vi "0805_Visão_de_máquina.vi"() -> ()   [LabVIEW 2017]
uses:
  <vilib>/userdefined/High Color/IMAQdx.ctl
  <vilib>/vision/driver/IMAQdx.llb/IMAQdx Acquisition Mode.ctl
  <vilib>/vision/driver/IMAQdx.llb/IMAQdx Buffer Number Mode.ctl
  <vilib>/vision/Classification.llb/IMAQ Classifier Read Options.ctl
  <vilib>/vision/driver/NI_Vision_Acquisition_Software.lvlib
  <vilib>/vision/NI_Vision_Development_Module.lvlib
panel:
  out "Array de classes":string[](array[string])
  out "Array de pos":string[](array[string])
  out "Array (0)":string[](array[string])
  out "Peça a ser manufatruada(0)":string[](array[string])
  out "Peça a ser manufatruada":string[](array[string])
  in  "Peça a ser manufaturada":T1
  out "x .and. y? 2":bool
  out "x = y? 2":bool
  out "x = y?":bool
  out "Boolean 2":bool
  out "concatenated string 3":string
  out "seletou_detectou":bool
  in  "Comunicação de dados":bool
  out "concatenated string 2":string
  out "concatenated string":string
  out "Boolean":bool
  out "Parar_esteira":bool
  out "aux":bool
  out "normal":u32
  out "parou":u32
  out "detectou":u32
  out "Detectou":bool
  out "reconheceu":bool
  out "bool_parou":bool
  out "bool_normal":bool
  out "bool_detectou":bool
  out "reconhecendo":bool
  out "Stop 3":bool
  out "seletor":enum16{"normal", "detectou", "parou"}(ring)=enum."detectou"
  in  "enum":enum16{"normal", "detectou", "parou"}(ring)=enum."detectou"
  out "x .and. y?":bool
  in  "dimensão_x_ROI_esteira":sgl=30.0
  in  "dimensão_y_ROI_esteira":sgl=30.0
  in  "posicao_y_ROI_esteira":sgl
  in  "posicao_x_ROI_esteira":sgl
  out "Local destino":T2(ring)
  in  "Tab Control":T3(tab)
  in  "Cluster A":T4
  in  "Cluster B":T4
  in  "Cluster C":T4
  in  "QRCode":bool
  out "Table":string[][](table)
  in  "Stop 2":bool
  in  "Stop 1":bool
  out "Imagem Original":T5(plugin-control)
  in  "Câmera":T6="cam1"
  out "XY Graph 2":cluster{"X":dbl, "Y":dbl}[](graph)
  # "ROTINA DE VISÃO COMPUTACIONAL"
  # "HISTÓRICO DE RECONHECIMENTO"
  # "DEFINI敲O DA ROI DA ESTEIRA"
  # "IMAGEM OBTIDA PELA CÂMERA"
  # "POSI敲O X"
  # "-100"
  # "POSI敲O Y"
  # "-254"
  # "DIMENSÃO X"
  # "84"
  # "DIMENSÃO Y"
  # "250"
  # "DEFINI敲O DOS LOCAIS DE DESTINO\nDA MANIPULA敲O"
  # "LOCAL DE DESTINO"
  # "Debug do reconhecimento"
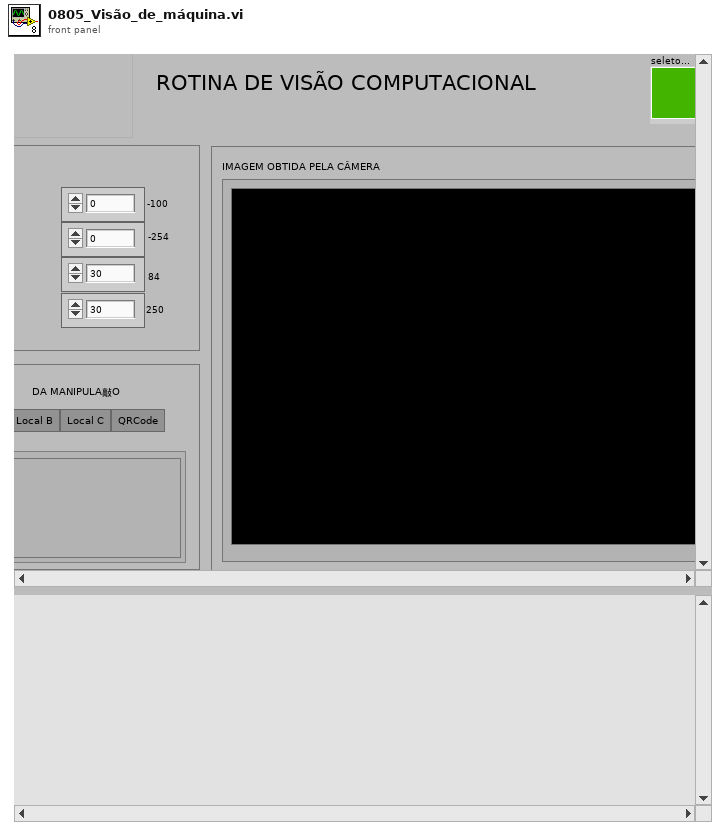
[diagram p1: front panel]
types:
  T1 = cluster{"Quadrado":bool, "Quadrado 2":bool, "Quadrado 3":bool}
  T2 = enum16{"Local A", "Local B", "Local C", "Discard"}
  T3 = enum32{"Local A", "Local B", "Local C", "QRCode"}
  T4 = cluster{"Quadrado":bool, "Triângulo":bool, "Trapézio":bool}
  T5 = typedef "IMAQ Image.ctl" = refnum<image>
  T6 = typedef "IMAQdx.ctl" = refnum<k21>
  T7 = typedef "NI_Vision_Acquisition_Software.lvlib/IMAQdx Acquisition Mode.ctl" = enum32{"One Shot", "Continuous"}
  T8 = typedef "NI_Vision_Acquisition_Software.lvlib/IMAQdx Buffer Number Mode.ctl" = enum32{"Next", "Last", "Buffer Number", "Every", "Last New"}
  T9 = cluster{"Global Rectangle":i32[], "Contours":cluster{"Contour Type":u32, "ROI Type":u32, "Points":i32[]}[]}
  T10 = typedef "ROI Descriptor" = cluster{"Global Rectangle":i32[], "Contours":cluster{"ID":enum32{"External", "Internal"}, "Type":u32, "Coordinates":i32[]}[]}
  T11 = typedef "IMAQ Classifier Read Options.ctl" = i32
  T12 = typedef "IMAQ Classifier Session.ctl" = refnum<k1>
  T13 = enum16{"Local A", "Local B", "Local C", "Discard"}[]
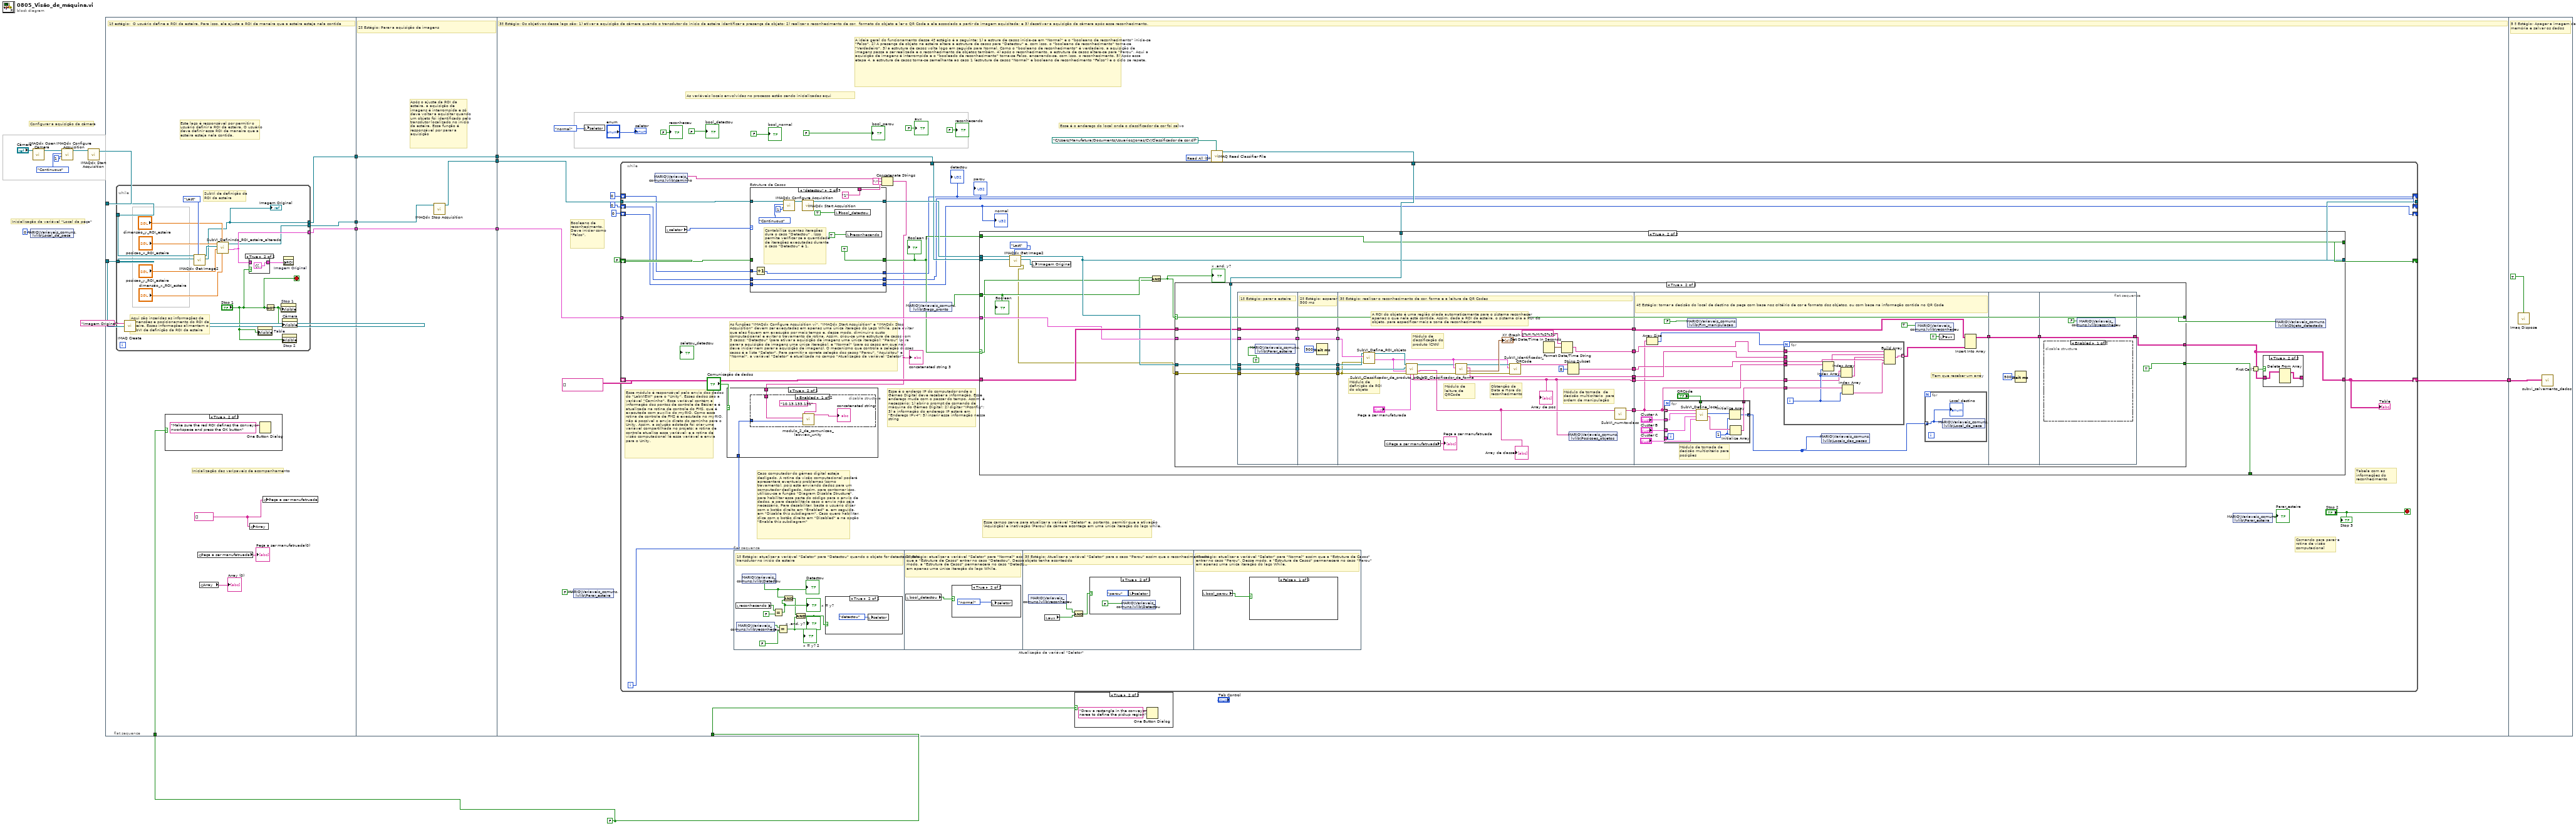
[diagram p0: block diagram]
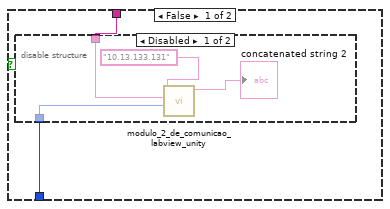
[diagram p4: hidden frame]
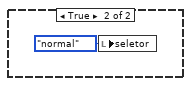
[diagram p10: hidden frame]
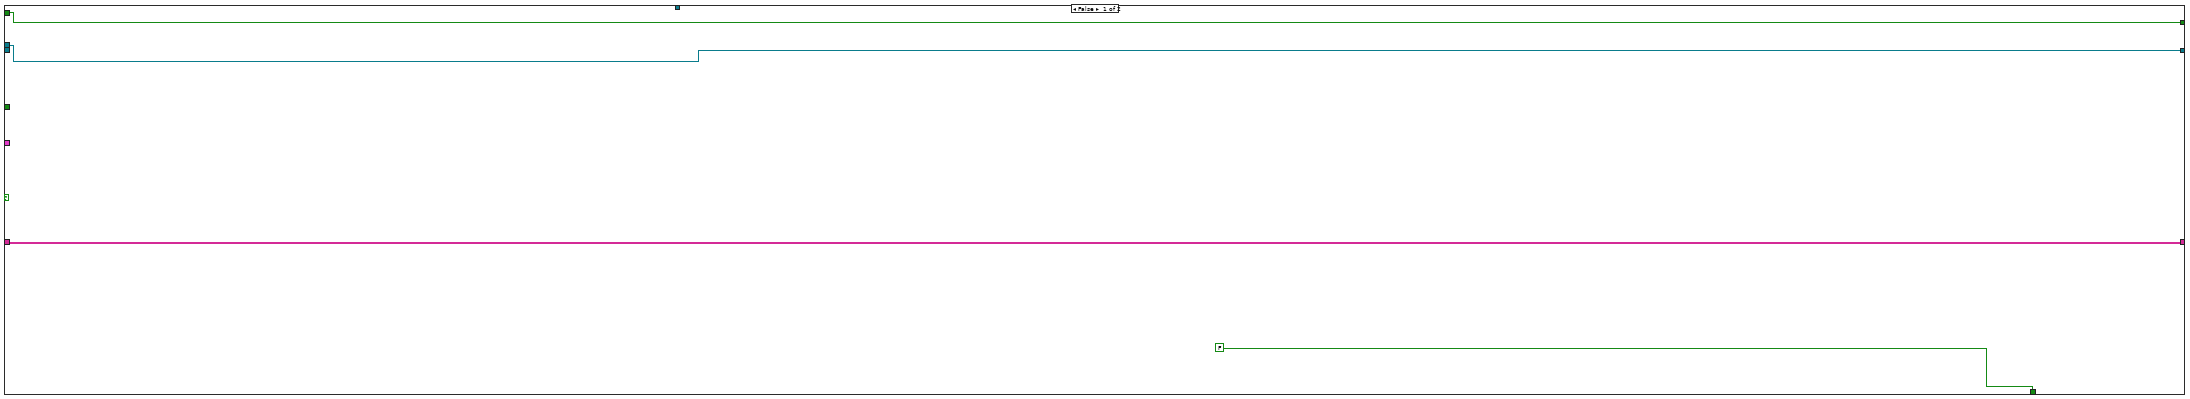
[diagram p11: hidden frame]
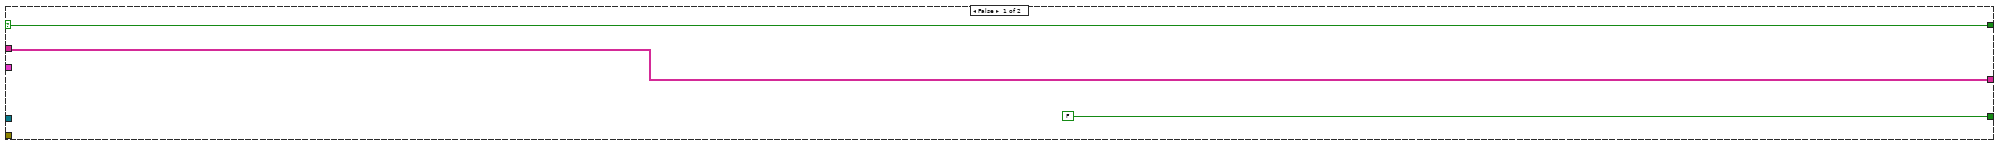
[diagram p13: hidden frame]
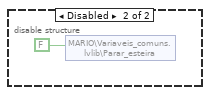
[diagram p14: hidden frame]
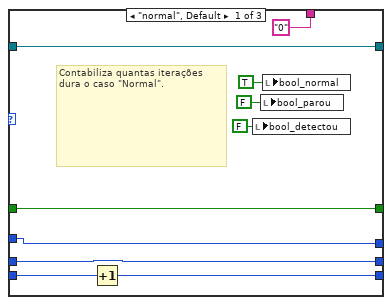
[diagram p15: hidden frame]
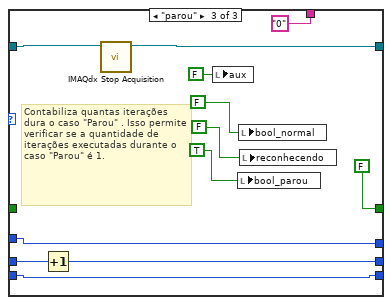
[diagram p16: hidden frame]
diagram:
  w10 = FALSE
  # "Inicialização da variável \"Local da peça\""
  # "Configurar a aquisição da câmera"
  n1 = shared-variable "MARIO\\Variaveis_comuns.lvlib\\Local_da_peca"(i8 0 ("Local_da_peca")) -> ()  [unwired: 1 in, 1 out]
  n2 = call <vilib>:"IMAQdx Open Camera.vi"("Session In"="Câmera") -> ("Session Out"=w17:T6)  [unwired: 9 in, 1 out]
  n3 = call <vilib>:"IMAQdx Configure Acquisition.vi"("Number of Buffers"=u32 1, "Continuous?"=IMAQdx_Acquisition_Mode."Continuous", "Session In"=w17) -> ("Session Out"=w16:T6)  [unwired: 7 in, 1 out]
  n4 = call <vilib>:"IMAQdx Start Acquisition.vi"("Session In"=w16) -> ("Session Out"=w7:T6)  [unwired: 9 in, 1 out]
  n5 = flat-sequence {
    tunnel: w7 -> [w26]
    tunnel: w11 -> [w25]
    tunnel: [w24] -> w4
    tunnel: [w23] -> w3
    tunnel: [w22] -> w2
    tunnel: w10 -> [w21]
    tunnel: w4 -> [w46]
    tunnel: w3 -> [w47]
    tunnel: [w47] -> w9
    tunnel: [w45] -> w8
    tunnel: w2 -> [w45]
    tunnel: [w44] -> w6
    tunnel: w9 -> [w65]
    tunnel: w10 -> [w69]
    tunnel: w8 -> [w62]
    tunnel: w6 -> [w60]
    tunnel: [w48] -> w1
    tunnel: w1 -> [w297]
    frame #0 {
      w18 = string[] []
      # "Inicialização das varipaveis de acompanhamento"
      # "Este laço é responsável por permitir o usuário definir a ROI da esteira. O usuário deve definir essa ROI de maneira que a esteira esteja nela contida."
      # "1º estágio:  O usuário define a ROI da esteira. Para isso, ele ajusta a ROI de maneira que a esteira esteja nela contida"
      n6 = while {
        tunnel: w26 -> [w40]
        tunnel: w25 -> [w39]
        tunnel: [w29] -> w24
        tunnel: [w30] -> w23
        tunnel: [w28] -> w22
        stop <- "Stop 1" stop-if-true
        # "SubVi de definição da ROI da esteira"
        # "Aqui são inseridas as informações de dimensões e posicionamento do ROI da esteira. Essas informações alimentam o SubVI de definição da ROI da esteira"
        n7 = call <vilib>:"IMAQdx Get Image2.vi"("Buffer Number Mode (Next)"=IMAQdx_Buffer_Number_Mode."Last", "Image In"=w39, "Session In"=w40) -> ("Image Out"=w28:T5, "Session Out"=w31:T6)  [unwired: 5 in, 2 out]
        "Imagem Original" <- w28
        n8 = call "SubVI_Definindo_ROI_esteira_alterado.vi"("largura_y"="dimensão_x_ROI_esteira", "largura_x"="dimensão_y_ROI_esteira", "ofset y"="posicao_y_ROI_esteira", "Session in"=w31, "ofset x"="posicao_x_ROI_esteira") -> ("ROI Descriptor"=w30:T10, "Session Out"=w29:T6)  [unwired: 4 in, 1 out]
        n9 = case shown="True" "Stop 1" {
          tunnel: w30 -> [w42 _]
          tunnel: [w42 T9 {"Global Rectangle"=[0, 0, 1, 1], "Contours"=[{"Contour Type"=0, "ROI Type"=1, "Points"=[0, 0]}]} ("ROI")] -> w38
          frame False {
          }
          frame True {
          }
        }
        n10 = property on="Table" class="Tbl (strict)"("Visible"="Stop 1") -> ()  [unwired: 2 in, 2 out]
        n11 = Not(x="Stop 1") -> (.not. x?=w37:bool)
        n12 = property on="Stop 1" class="Bool"("Visible"=w37) -> ()  [unwired: 2 in, 2 out]
        n13 = property on="Stop 2" class="Bool"("Visible"="Stop 1") -> ()  [unwired: 2 in, 2 out]
        n14 = property on="Câmera" class="IMAQdx (strict)"("Visible"=w37) -> ()  [unwired: 2 in, 2 out]
        n15 = property on="Imagem Original" class="ImageControl"("ROI"=w38) -> ()  [unwired: 2 in, 2 out]
      }
      n16 = case shown="True" w21 {
        frame False {
        }
        frame True {
          n17 = One Button Dialog(message="Make sure the red ROI defines the conveyor \nworkspace and press the OK button") -> ()  [unwired: 1 in, 1 out]
        }
      }
      n18 = global read "Peça_manufaturada-acompanhamento.vi" "Peça a ser manufatruada"() -> (→"Peça a ser manufatruada(0)":string[])
      n19 = global read "Pçea_x-atual.vi" "Array"() -> (→"Array (0)":string[])
      n20 = global write "Pçea_x-atual.vi" "Array"(w18) -> ()
      n21 = global write "Peça_manufaturada-acompanhamento.vi" "Peça a ser manufatruada"(w18) -> ()
    }
    frame #1 {
      # "Após o ajuste da ROI da esteira, a aquisição de imagens é interrompida e só deve voltar a aquisitar quando um objeto foi identificado pelo transdutor localizado no início da esteira. Essa função é responsável por parar a aquisição"
      # "2º Estágio: Parar a aquisição de imagens"
      n22 = call <vilib>:"IMAQdx Stop Acquisition.vi"("Session In"=w46) -> ("Session Out"=w44:T6)  [unwired: 9 in, 1 out]
    }
    frame #2 {
      w68 = T11 0 items=["Read All", "Add Samples, Do Not Change Options", "Read Options, Do Not Add Samples"] ("Read Options")
      # "Esse é o endereço do local onde o classificador de cor foi salvo"
      # "A ideia geral do funcionamento desse 4º estágio é a seguinte: 1) a estrura de casos inicia-se em \"Normal\" e o \"booleano de reconhecimento\" inicia-se \"Falso\". 2) A presença de objeto na esteira altera a estrutura de casos para \"Detectou\" e, com isso, o \"booleano de reconhecimento\" torna-se \"Verdadeiro\". 3) a estrutura de casos volta logo em seguida para Normal. Como o \"booleano de reconhecimento\" é verdadeiro, a aquisição de imagens passa a ser realizada e o reconhecimento de objetos também. 4) após o reconhecimento, a estrutura de casos altera-se para \"Parou\". Aqui a aquisição de imagens é interrompida e o \"booleado de reconhecimento\" torna-se Falso, encerrando-se, com isso, o reconhecimento. 5) Após essa etapa 4, a estrutura de casos torna-se semelhante ao caso 1 (estrutura de casos \"Normal\" e booleano de reconhecimento \"Falso\") e o ciclo se repete."
      # "As variáveis locais envolvidas no processo estão sendo inicializadas aqui"
      # "Booleano de reconhecimento. Deve iniciar como \"Falso\"."
      # "3º Estágio: Os objetivos desse laço são: 1) ativar a aquisição da câmera quando o transdutor do início da esteira identificar a presença de objeto; 2) realizar o reconhecimento de cor,  formato do objeto e ler o QR Code a ele associado a partir da imagem aquisitada; e 3) desativar a aquisição da câmera após esse reconhecimento."
      n23 = shared-variable "MARIO\\Variaveis_comuns.lvlib\\Parar_esteira"(FALSE ("Parar_esteira")) -> ()  [unwired: 1 in, 1 out]
      n24 = local write "seletor"(enum16{"normal", "detectou", "parou"}."normal") -> ()
      n25 = case shown="True" w69 {
        frame False {
        }
        frame True {
          n26 = One Button Dialog(message="Draw a rectangle in the conveyor\narea to define the pickup region") -> ()  [unwired: 1 in, 1 out]
        }
      }
      n27 = call "IMAQ Read Classifier File"("File Path"=path "C:/Users/Manufatura/Documents/Usuarios/Jonas/CV/Classificador de cor.clf", "Read Options"=w68) -> ("Classifier Session"=w67:T12)  [unwired: 2 in, 7 out]
      n28 = while {
        tunnel: w65 -> [w95]
        tunnel: w67 -> [w96]
        shift-right: [w76] -> w48
        shift-left: string[][] [] ("Table") -> [w77]
        tunnel: w62 -> [w93]
        shift-right: [w90] -> _
        shift-left: FALSE -> [w92]
        tunnel: w60 -> [w88]
        tunnel: [w89] -> _
        shift-right: [w84] -> _
        shift-left: u32 0 ("Number of Buffers") -> [w81]
        shift-right: [w83] -> _
        shift-left: u32 0 ("Number of Buffers") -> [w80]
        shift-right: [w82] -> _
        shift-left: u32 0 ("Number of Buffers") -> [w79]
        i -> [w71]
        stop <- "Stop 2" stop-if-true
        # "Tabela com as informações do reconhecimento"
        # "Comando para parar a rotina de visão computacional"
        # "Esse campo serve para atualizar a variável \"Seletor\" e, portanto, permitir que a ativação (Aquisição) e inativação (Parou) da câmera aconteça em uma única iteração do laço while."
        # "Esse é o enderço IP do computador onde o Gêmeo Digital deve receber a informação. Esse endereço muda com o passar do tempo. Assim, é necessário: 1) abrir o prompt de comando da máquina do Gêmeo Digital; 2) digitar \"IPconfig\"; 3) a informação do endereço IP estará em \"Endereço IPv4\"; 5) inserir essa informação nessa string"
        # "Caso computador do gêmeo digital esteja desligado, A rotina de visão computacional poderá apresentará eventuais problemas (como travamento), pois está enviando dados para um computador desligado. Assim, para contornar isso, utilizou-se a função \"Diagram Disable Structure\", para habilitar essa parte do código para o envio de dados, e para desabilitá-la caso o envio não seja necessário. Para desabilitar, basta o usuário clicar com o botão direito em \"Enabled\" e, em seguida, em \"Disable this subdiagram\". Caso quero habilitar, clica com o botão direito em \"Disabled\" e na opção \"Enable this subdiagram\""
        # "Esse módulo é responsável pelo envio dos dados do \"LabVIEW\" para o \"Unity\". Esses dados são a variável \"Caminho\". Essa variável contém a informação dos pontos de controle de Bézier e é atualizada na rotina de controle do FMS, que é executada com auxílio do myRIO. Como essa rotina de controle de FMS é executada no myRIO, não é possível o envio direto do caminho para o Unity. Assim, a solução adotada foi criar uma  variável compartilhada no projeto: a rotina de controle atualiza essa variável; e a rotina de visão computacional lê essa variável e envia para o Unity."
        # "As funções \"IMAQdx Configure Acquisition vi\", \"IMAQdx Start Acquisition\" e \"IMAQdx Stop Acquisition\" devem ser executadas em apenas uma única iteração do Laço While, para evitar que elas fiquem em execução por mais tempo e, desse modo, diminuir o custo computacioanal e evitar o travamento da rotina. Assim, criou-se uma estrutura de casos com 3 casos: \"Detectou\" (para ativar a aquisição de imagens uma única iteração); \"Parou\" (para parar a aquisição de imagens uma única iteração), e \"Normal\" (para os casos em que não deve iniciar nem parar a aquisição de imagens). O mecanismo que controla a seleção desses casos é a lista \"Seletor\". Para permitir a correta seleção dos casos \"Parou\", \"Aquisitou\" e \"Normal\", a variável \"Seletor\" é atualizada no campo \"Atualização da variável 'Seletor'\""
        n29 = shared-variable "MARIO\\Variaveis_comuns.lvlib\\caminho"() -> (w74:string)  [unwired: 1 in, 1 out]
        n30 = local read "seletor"() -> (w85:enum16{"normal", "detectou", "parou"})
        n31 = flat-sequence "Atualização da variável \"Seletor\"" {
          frame #0 {
            # "1º Estágio: atualizar a variável \"Seletor\" para \"Detectou\" quando o objeto for detectado pelo transdutor no início da esteira"
            n32 = local read "reconhecendo"() -> (w113:bool)
            n33 = shared-variable "MARIO\\Variaveis_comuns.lvlib\\reconheceu"() -> (w115:bool)  [unwired: 1 in, 1 out]
            n34 = shared-variable "MARIO\\Variaveis_comuns.lvlib\\Detectou"() -> (w109:bool)  [unwired: 1 in, 1 out]
            "Detectou" <- w109
            n35 = Equal?(x=w113, y=FALSE) -> (x = y?=w114:bool)
            "x = y?" <- w114
            n36 = Equal?(x=w115, y=FALSE) -> (x = y?=w116:bool)
            "x = y? 2" <- w116
            n37 = And(x=w109, y=w114) -> (x .and. y?=w112:bool)
            n38 = And(x=w112, y=w116) -> (x .and. y?=w117:bool)
            "x .and. y? 2" <- w117
            n39 = case shown="True" w117 {
              frame False {
              }
              frame True {
                n40 = local write "seletor"(enum16{"normal", "detectou", "parou"}."detectou") -> ()
              }
            }
          }
          frame #1 {
            # "2º Estágio: atualizar a variável \"Seletor\" para \"Normal\" assim que a \"Estrutura de Casos\" entrar no caso \"Detectou\". Desse modo, a \"Estrutura de Casos\" permanecerá no caso \"Detectou\" em apenas uma única iteração do laço While."
            n41 = local read "bool_detectou"() -> (w119:bool)
            n42 = case shown="True" w119 {
              frame False {
              }
              frame True {
                n43 = local write "seletor"(enum16{"normal", "detectou", "parou"}."normal") -> ()
              }
            }
          }
          frame #2 {
            # "3º Estágio: Atualizar a variável \"Seletor\" para o caso \"Parou\" assim que o reconhecimento do objeto tenha acontecido"
            n44 = shared-variable "MARIO\\Variaveis_comuns.lvlib\\reconheceu"() -> (w123:bool)  [unwired: 1 in, 1 out]
            n45 = local read "aux"() -> (w122:bool)
            n46 = And(x=w123, y=w122) -> (x .and. y?=w121:bool)
            n47 = case shown="True" w121 {
              frame False {
              }
              frame True {
                n48 = shared-variable "MARIO\\Variaveis_comuns.lvlib\\Detectou"(FALSE ("Detectou")) -> ()  [unwired: 1 in, 1 out]
                n49 = local write "seletor"(enum16{"normal", "detectou", "parou"}."parou" ("lista")) -> ()
              }
            }
          }
          frame #3 {
            # "4º estágio: atualizar a variável \"Seletor\" para \"Normal\" assim que a \"Estrutura de Casos\" entrar no caso \"Parou\". Desse modo, a \"Estrutura de Casos\" permanecerá no caso \"Parou\" em apenas uma única iteração do laço While."
            n50 = local read "bool_parou"() -> (w126:bool)
            n51 = case shown="False" w126 {
              frame False {
              }
              frame True {
                n52 = local write "seletor"(enum16{"normal", "detectou", "parou"}."normal" ("lista")) -> ()
              }
            }
          }
        }
        n53 = case "Estrutura de Casos" shown="\"detectou\"" w85 {
          tunnel: [w269 w279 w294] -> w94
          tunnel: w88 -> [w269 w280 w295]
          tunnel: [w270 TRUE FALSE] -> w91
          tunnel: w92 -> [w270 _ _]
          tunnel: w81 -> [w264 w275 w287]
          tunnel: w80 -> [w263 w273 w289]
          tunnel: w79 -> [w265 w272 w286]
          tunnel: [w264 w274 w287] -> w84
          tunnel: [w263 w273 w288] -> w83
          tunnel: [w262 w272 w286] -> w82
          tunnel: ["0" ("string") "1" ("string") "0" ("string")] -> w72
          frame "normal", Default {
            # "Contabiliza quantas iterações dura o caso \"Normal\"."
            n54 = Increment(x=w265) -> (x+1=w262:u32)
            n55 = local write "bool_detectou"(FALSE ("detectou")) -> ()
            n56 = local write "bool_parou"(FALSE ("bool_parou")) -> ()
            n57 = local write "bool_normal"(TRUE ("bool_normal")) -> ()
          }
          frame "detectou" {
            # "Contabiliza quantas iterações dura o caso \"Detectou\" . Isso permite verificar se a quantidade de iterações executadas durante o caso \"Detectou\" é 1."
            n58 = Increment(x=w275) -> (x+1=w274:u32)
            n59 = call <vilib>:"IMAQdx Configure Acquisition.vi"("Number of Buffers"=u32 1, "Continuous?"=IMAQdx_Acquisition_Mode."Continuous", "Session In"=w280) -> ("Session Out"=w281:T6)  [unwired: 7 in, 1 out]
            n60 = call <vilib>:"IMAQdx Start Acquisition.vi"("Session In"=w281) -> ("Session Out"=w279:T6)  [unwired: 9 in, 1 out]
            n61 = local write "bool_detectou"(TRUE ("bool_detectou")) -> ()
            n62 = local write "reconhecendo"(TRUE ("reconhecendo")) -> ()
          }
          frame "parou" {
            # "Contabiliza quantas iterações dura o caso \"Parou\" . Isso permite verificar se a quantidade de iterações executadas durante o caso \"Parou\" é 1."
            n63 = Increment(x=w289) -> (x+1=w288:u32)
            n64 = call <vilib>:"IMAQdx Stop Acquisition.vi"("Session In"=w295) -> ("Session Out"=w294:T6)  [unwired: 9 in, 1 out]
            n65 = local write "aux"(FALSE ("aux")) -> ()
            n66 = local write "bool_parou"(TRUE ("bool_parou")) -> ()
            n67 = local write "bool_normal"(FALSE ("bool_normal")) -> ()
            n68 = local write "reconhecendo"(FALSE ("reconhecendo")) -> ()
          }
        }
        "detectou" <- w84
        "parou" <- w83
        "normal" <- w82
        "Boolean 2" <- w91
        n69 = Concatenate Strings(w74, ";" ("string"), w72) -> (w70:string)
        "concatenated string 3" <- w70
        n70 = case shown="True" "Comunicação de dados" {
          tunnel: w71 -> [w98 w104]
          tunnel: w70 -> [w97 w103]
          frame False {
            n71 = disable-structure shown="Disabled" {
              disable-tunnel: w98 -> [w100 _]
              disable-tunnel: w97 -> [w99 _]
              frame Disabled {
                n72 = call "modulo_2_de_comunicao_labview_unity.vi"("number"=w100, "String"=w99, "address"="10.13.133.131") -> ("concatenated string"=→"concatenated string 2":string)  [unwired: 7 in, 1 out]
              }
              frame Enabled {
              }
            }
          }
          frame True {
            n73 = disable-structure shown="Enabled" {
              disable-tunnel: w104 -> [w106 _]
              disable-tunnel: w103 -> [w105 _]
              frame Enabled {
                n74 = call "modulo_2_de_comunicao_labview_unity.vi"("number"=w106, "String"=w105, "address"="10.13.133.131") -> ("concatenated string"=→"concatenated string":string)  [unwired: 7 in, 1 out]
              }
              frame Disabled {
              }
            }
          }
        }
        n75 = shared-variable "MARIO\\Variaveis_comuns.lvlib\\Braço_pronto"() -> (w87:bool)  [unwired: 1 in, 1 out]
        n76 = case shown="True" w91 {
          selector: w91 -> [_ w135]
          tunnel: w96 -> [_ w148]
          tunnel: w77 -> [w131 w147]
          tunnel: [w131 w132] -> w76
          tunnel: w95 -> [_ w144]
          tunnel: w94 -> [w129 w141]
          tunnel: w93 -> [_ w140]
          tunnel: [w130 w138] -> w90
          tunnel: w91 -> [w130 w138]
          tunnel: [w129 w139] -> w89
          tunnel: w87 -> [_ w136]
          tunnel: [FALSE w137] -> _
          frame False {
          }
          frame True {
            n77 = call <vilib>:"IMAQdx Get Image2.vi"("Buffer Number Mode (Next)"=IMAQdx_Buffer_Number_Mode."Last", "Image In"=w140, "Session In"=w141) -> ("error out"=w133:errorcluster, "Image Out"=w142:T5, "Session Out"=w139:T6)  [unwired: 5 in, 1 out]
            n78 = local write "Imagem Original"(w142) -> ()
            n79 = And(x=w136, y=w135) -> (x .and. y?=w134:bool)
            "x .and. y?" <- w134
            n80 = case shown="True" w134 {
              selector: w134 -> [w153 w175]
              tunnel: w139 -> [_ w178]
              tunnel: w148 -> [_ w180]
              tunnel: w133 -> [_ w179]
              tunnel: [w154 w177] -> w132
              tunnel: w147 -> [w154 w176]
              tunnel: [w153 w175] -> w145
              tunnel: w144 -> [_ w174]
              tunnel: [FALSE TRUE] -> w137
              frame False {
              }
              frame True {
                n81 = flat-sequence {
                  tunnel: w176 -> [w183]
                  tunnel: w178 -> [w184]
                  tunnel: w179 -> [w185]
                  tunnel: w180 -> [w186]
                  tunnel: [w186] -> w173
                  tunnel: [w185] -> w171
                  tunnel: [w184] -> w169
                  tunnel: [w183] -> w167
                  tunnel: w174 -> [w182]
                  tunnel: [w182] -> w165
                  tunnel: w173 -> [w192]
                  tunnel: [w192] -> w172
                  tunnel: w171 -> [w191]
                  tunnel: [w191] -> w170
                  tunnel: w169 -> [w190]
                  tunnel: [w190] -> w168
                  tunnel: w167 -> [w189]
                  tunnel: [w189] -> w166
                  tunnel: w165 -> [w188]
                  tunnel: [w188] -> w164
                  tunnel: w172 -> [w202]
                  tunnel: w170 -> [w201]
                  tunnel: w168 -> [w210]
                  tunnel: w166 -> [w208]
                  tunnel: w164 -> [w211]
                  tunnel: [w208] -> w163
                  tunnel: [w205] -> w159
                  tunnel: [w204] -> w158
                  tunnel: [w203] -> w157
                  tunnel: [w193] -> w156
                  tunnel: [w196] -> w155
                  tunnel: w163 -> [w233]
                  tunnel: [w230] -> w161
                  tunnel: w159 -> [w224]
                  tunnel: w158 -> [w223]
                  tunnel: w157 -> [w222]
                  tunnel: w156 -> [w221]
                  tunnel: w155 -> [w219]
                  tunnel: w161 -> [w257]
                  tunnel: [w257] -> w160
                  tunnel: [w259] -> w177
                  tunnel: w160 -> [w259]
                  frame #0 {
                    # "1º Estágio: parar a esteira"
                    n82 = shared-variable "MARIO\\Variaveis_comuns.lvlib\\Parar_esteira"(TRUE ("Parar_esteira")) -> ()  [unwired: 1 in, 1 out]
                  }
                  frame #1 {
                    # "2º Estágio: esperar 500 ms"
                    n83 = Wait (ms)(milliseconds to wait=u32 900) -> ()  [unwired: 1 out]
                  }
                  frame #2 {
                    # "Módulo de tomada  de decisão multicritério  para ordem de manipulação"
                    # "A ROI do objeto é uma região criada automaticamente para o sistema reconhecer apenas o que nela está contida. Assim, dada a ROI da esteira, o sistema cria a ROI do objeto, para especificar mais a zona de reconhecimento"
                    # "Módulo de definição da ROI do objeto"
                    # "Módulo de classificação do produto (CNN)"
                    # "Módulo de leitura de QRCode"
                    # "Obtenção da Data e Hora do reconhecimento"
                    # "3º Estágio: realizar o reconhecimento de cor, forma e a leitura de QR Codes"
                    n84 = call "SubVI_Define_ROI_objeto.vi"("error in (no error)"=w201, "ROI Esteira"=w211, "Session In"=w210) -> ("ROI Objeto"=w200:T10, "Session Out"=w209:T6)  [unwired: 5 in, 2 out]
                    n85 = global read "Peça_manufaturada-acompanhamento.vi" "Peça a ser manufatruada"() -> (→"Peça a ser manufatruada":string[])
                    n86 = call "SubVI_Classificador_de_produto_cnn_v2.vi"("Peça a ser manufaturada"="Peça a ser manufaturada", "error in"=w201, "ROI Objeto"=w200, "Classifier Session"=w202, "Session In"=w209) -> ("error out"=w199:errorcluster, "Array_out"=w194:string[], "Session Out"=w198:T6, "Array 2"=w193:string[])  [unwired: 2 in]
                    "Array de pos" <- w193
                    "Array de classes" <- w194
                    n87 = call "SubVI_Classificador_de_forma.vi"("error in"=w199, "ROI Objeto"=w200, "Session In"=w198) -> ("error out"=w214:errorcluster, "Points"=→"XY Graph 2":cluster{"X":dbl, "Y":dbl}[], "Forma"=w204:string, "Session Out"=w206:T6)  [unwired: 5 in]
                    n88 = call "SubVI_Identificador_QRCode.vi"("error in"=w214, "ROI Objeto"=w200, "Session In"=w206) -> ("Data"=w213:string)  [unwired: 7 in, 1 out]
                    n89 = Get Date/Time In Seconds() -> (seconds since 1Jan1904=w215:timestamp)
                    n90 = Format Date/Time String(time format string (%c)="%H:%M:%S%3u", seconds (now)=w215) -> (date/time string=w205:string)  [unwired: 1 in]
                    n91 = String Subset(string=w213, offset (0)=8) -> (substring=w203:string)  [unwired: 1 in]
                    n92 = shared-variable "MARIO\\Variaveis_comuns.lvlib\\Posicoes_objetos"(w193) -> ()  [unwired: 1 in, 1 out]
                    n93 = call "SubVI_num-to-class.vi"("Array in"=w194) -> ("Array out"=w196:string[])  [unwired: 10 in]
                  }
                  frame #3 {
                    # "Tem que receber um array"
                    # "Módulo de tomada de decisão multicritério para posições"
                    # "4º Estágio: tomar a decisão do local de destino da peça com base nos critéirio de cor e formato dos objetos, ou com base na informação contida no QR Code"
                    n94 = Array Size(array=w219) -> (size(s)=w226:i32)
                    n95 = for {
                      tunnel: "QRCode" -> [w255]
                      tunnel: w219 -> [w254] mode=indexing
                      tunnel: "Cluster A" -> [w253]
                      tunnel: "Cluster B" -> [w252]
                      tunnel: "Cluster C" -> [w251]
                      tunnel: [w249] -> w220 mode=concatenating
                      tunnel: [w246] -> w218 mode=concatenating
                      w248 = 1 ("dimension size")
                      n96 = call "SubVI_Define_local.vi"("QRCode"=w255, "Cluster C"=w251, "Cluster B"=w252, "Cluster A"=w253, "Class"=w254) -> ("Destino"=w250:string, "Local destino"=w247:T2)  [unwired: 5 in]
                      n97 = Initialize Array(w247, w248) -> (w246:T13)
                      n98 = Initialize Array(w250, w248) -> (w249:string[])
                    }
                    n99 = shared-variable "MARIO\\Variaveis_comuns.lvlib\\Fim_manipulacao"(FALSE) -> ()  [unwired: 1 in, 1 out]
                    n100 = for {
                      N: w226 -> [_]
                      tunnel: w224 -> [w245]
                      tunnel: w223 -> [_]
                      tunnel: [w244] -> w225 mode=indexing
                      tunnel: w219 -> [w243]
                      tunnel: w220 -> [w242]
                      tunnel: w222 -> [w241]
                      tunnel: w221 -> [w237]
                      i -> [w238]
                      n101 = Index Array(array=w243, index=w238) -> (element=w239:string)
                      n102 = Index Array(array=w237, index=w238) -> (element=w236:string)
                      n103 = Index Array(array=w242, index=w238) -> (element=w240:string)
                      n104 = Build Array(w245, w239, w236, w241, w240) -> (w244:string[])
                    }
                    n105 = shared-variable "MARIO\\Variaveis_comuns.lvlib\\Locais_das_pecas"(w218) -> ()  [unwired: 1 in, 1 out]
                    n106 = shared-variable "MARIO\\Variaveis_comuns.lvlib\\reconheceu"(TRUE ("reconheceu")) -> ()  [unwired: 1 in, 1 out]
                    n107 = for {
                      tunnel: w218 -> [w235] mode=indexing
                      n108 = shared-variable "MARIO\\Variaveis_comuns.lvlib\\Local_da_peca"(w235) -> ()  [unwired: 1 in, 1 out]
                      "Local destino" <- w235
                    }
                    n109 = local write "aux"(TRUE ("aux")) -> ()
                    n110 = Insert Into Array(array=w233, new element=w225) -> (w230:string[][])  [unwired: 2 in]
                  }
                  frame #4 {
                    n111 = Wait (ms)(milliseconds to wait=u32 500) -> ()  [unwired: 1 out]
                  }
                  frame #5 {
                    n112 = disable-structure shown="Enabled" {
                      frame Enabled {
                      }
                      frame Disabled {
                        n113 = shared-variable "MARIO\\Variaveis_comuns.lvlib\\Parar_esteira"(FALSE ("Parar_esteira")) -> ()  [unwired: 1 in, 1 out]
                      }
                    }
                    n114 = shared-variable "MARIO\\Variaveis_comuns.lvlib\\reconheceu"(FALSE ("reconheceu")) -> ()  [unwired: 1 in, 1 out]
                  }
                }
              }
            }
            n115 = First Call?() -> (First Call?: T/F=w146:bool)
            n116 = case shown="True" w146 {
              tunnel: w132 -> [w149 w151]
              tunnel: [w149 w150] -> _
              frame False {
              }
              frame True {
                n117 = Delete From Array(array=w151) -> (array with subset deleted=w150:string[][])  [unwired: 3 in, 1 out]
              }
            }
            n118 = shared-variable "MARIO\\Variaveis_comuns.lvlib\\Objeto_detectado"(w145) -> ()  [unwired: 1 in, 1 out]
            "Boolean" <- w136
          }
        }
        "Table" <- w76
        n119 = shared-variable "MARIO\\Variaveis_comuns.lvlib\\Parar_esteira"() -> (→"Parar_esteira":bool)  [unwired: 1 in, 1 out]
        "Stop 3" <- "Stop 2"
      }
      "reconhecendo" <- FALSE ("reconheceu")
      "seletor" <- "enum"
      "bool_detectou" <- FALSE
      "bool_normal" <- FALSE
      "bool_parou" <- FALSE
      "reconheceu" <- FALSE ("reconheceu")
      "aux" <- FALSE
    }
    frame #3 {
      # "5 º Estágio: Apagar a imagem da memória e salvar os dados"
      n120 = call "Imaq Dispose"("All Images? (No)"=TRUE) -> ()  [unwired: 5 in, 1 out]
      n121 = call "subvi_salvamento_dados.vi"("Table"=w297) -> ()  [unwired: 10 in, 1 out]
    }
  }
  n122 = call "IMAQ Create"("Image Name"="Imagem Original") -> ("New Image"=w11:T5)  [unwired: 4 in, 1 out]
